vi "instance count allowed.vi"(8 "error in":errorcluster, 11 "FPGA Module configuration in":refnum<class "FPGA Module configuration.lvclass">) -> (0 "error out":errorcluster, 2 "instances allowed":i32, 3 "FPGA Module configuration out":refnum<class "FPGA Module configuration.lvclass">)   [LabVIEW 2017, in "FPGA Module configuration.lvclass"]
uses:
  FPGA Module configuration.lvclass
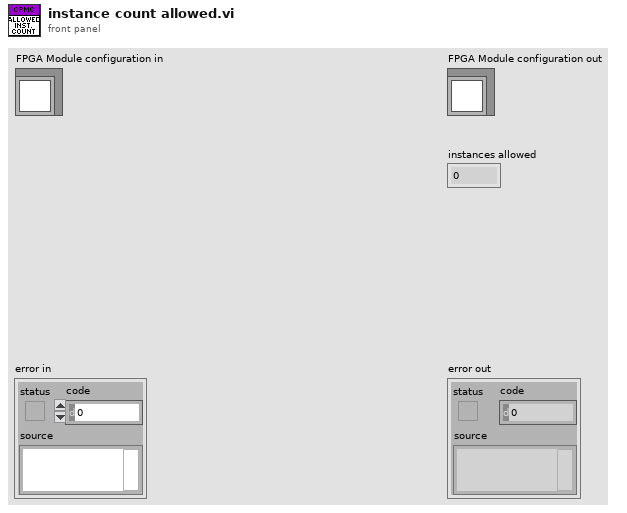
[diagram p1: front panel]
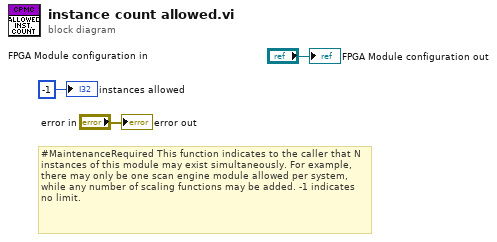
[diagram p0: block diagram]
diagram:
  # "#MaintenanceRequired This function indicates to the caller that N instances of this module may exist simultaneously. For example, there may only be one scan engine module allowed per system, while any number of scaling functions may be added. -1 indicates no limit."
  "error out" <- "error in"
  "FPGA Module configuration out" <- "FPGA Module configuration in"
  "instances allowed" <- -1 ("instances allowed")
